vi "CLPT_Piezo_Solver.vi"() -> ()   [LabVIEW 2012]
uses:
  LEM_Params.ctl
panel:
  out "Displacement Ratio":dbl
  in  "Stop Button":bool
  in  "Constants.P":dbl=-500.0
  in  "Constants.Vac":dbl=-10.0
  out "LEM Parameters":T1
  out "error out":errorcluster
  out "XY Graph":cluster{"Radius":dbl[], "W(r)":dbl[]}(graph)
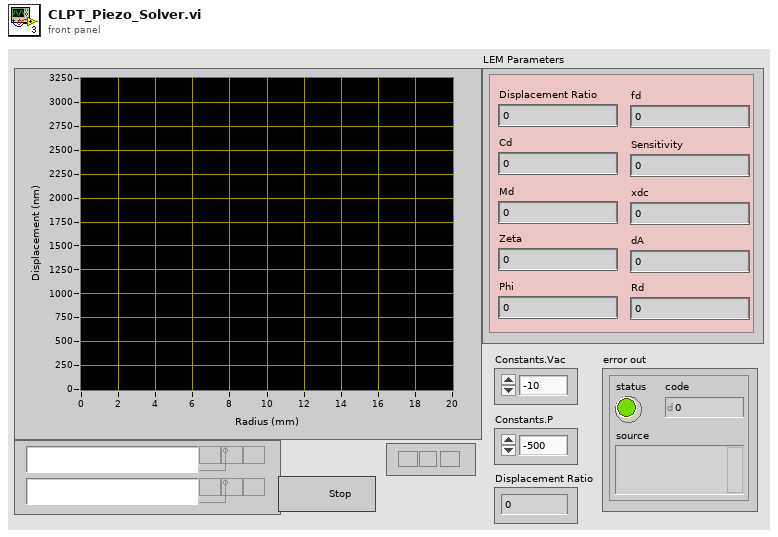
[diagram p1: front panel]
types:
  T1 = typedef "LEM_Params.ctl" = cluster{"Displacement Ratio":dbl, "Cd":dbl, "Md":dbl, "xdc":dbl, "fd":dbl, "Sensitivity":dbl, "dA":dbl, "Rd":dbl, "Zeta":dbl, "Phi":dbl}
  T2 = typedef "Model Data.ctl" = cluster{"Disc Properties":cluster{"Type":T3, "Disc Model":T4}, "Constants":cluster{"Radius":dbl[], "U(r)":dbl[], "W(r)":dbl[], "Vac":dbl, "P":dbl, "RiRo":dbl, "Area Density (r)":dbl[], "Ro":dbl, "Ri":dbl, "Z":dbl[], "Nr":dbl, "Mr":dbl, "c":dbl[], "AoC":dbl, "BoC":dbl, "AiC":dbl, "BiC":dbl, "f1":dbl, "f2":dbl}, "LEM Parameters":T1, "Layer Properties":T5[], "Matricies":T6}
  T3 = typedef "PZT type.ctl" = enum16{"Bimorph", "Unimorph"}
  T4 = typedef "Piezo_Discs.ctl" = enum16{"FTBD-21T-4.0A1", "PZT-5A (Gallas 1)", "PZT-5A (Gallas 2)", "AB4113B", "Create new disc...", "Load disc from file..."}
  T5 = typedef "Layer Properties.ctl" = cluster{"E":dbl, "R":dbl, "rho":dbl, "rhoA":dbl, "v":dbl, "A":dbl, "t":dbl, "d31":dbl, "size":enum16{"Outer", "Inner"}}
  T6 = typedef "Matricies.ctl" = cluster{"Aint":dbl[][], "Bint":dbl[][], "Dint":dbl[][], "Aout":dbl[][], "Bout":dbl[][], "Dout":dbl[][], "b":dbl[], "K":dbl[][]}
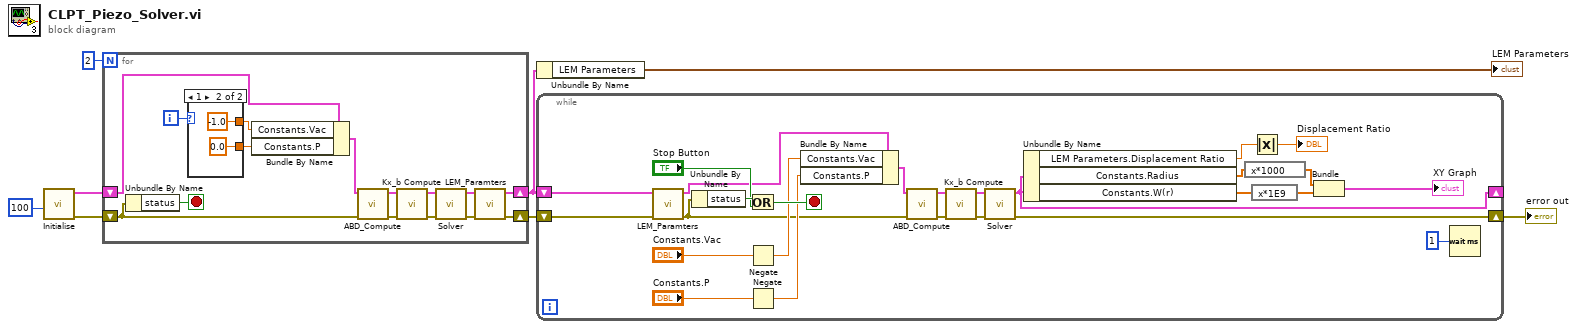
[diagram p0: block diagram]
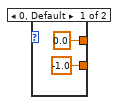
[diagram p2: hidden frame]
diagram:
  n1 = call "Initialise.vi"("Radial Points"=100) -> ("error out"=w5:errorcluster, "Model Data"=w7:T2)  [unwired: 9 in]
  n2 = for {
    N: 2 -> [_]
    shift-right: [w10] -> w2
    shift-left: w7 -> [w23]
    shift-right: [w15] -> w3
    shift-left: w5 -> [w9]
    i -> [w14]
    stop <- w11 stop-if-true
    n3 = Unbundle By Name(w9) -> ("status"=w11:bool)
    n4 = case shown="1" w14 {
      tunnel: [0.0 -1.0] -> w13
      tunnel: [-1.0 0.0] -> w12
      frame 0, Default {
      }
      frame 1 {
      }
    }
    n5 = Bundle By Name(cluster=w23, "Constants.Vac"=w13, "Constants.P"=w12) -> (w22:T2)
    n6 = call "ABD_Compute.vi"("error in"=w9, "Model Data"=w22) -> ("error out"=w21:errorcluster, "Model Data out"=w20:T2)  [unwired: 8 in]
    n7 = call "Kx_b Compute.vi"("error in"=w21, "Model Data"=w20) -> ("error out"=w19:errorcluster, "Model Data out"=w18:T2)  [unwired: 8 in]
    n8 = call "Solver.vi"("error in"=w19, "Model Data"=w18) -> ("error out"=w16:errorcluster, "Model Data out"=w17:T2)  [unwired: 8 in]
    n9 = call "LEM_Paramters.vi"("error in"=w16, "Model Data"=w17) -> ("error out"=w15:errorcluster, "Model Data Out"=w10:T2)  [unwired: 8 in]
  }
  n10 = Unbundle By Name(w2) -> ("LEM Parameters"=→"LEM Parameters":T1)
  n11 = while {
    shift-right: [w36] -> w4
    shift-left: w3 -> [w33]
    shift-right: [w43] -> _
    shift-left: w2 -> [w31]
    stop <- w39 stop-if-true
    n12 = call "LEM_Paramters.vi"("error in"=w33, "Model Data"=w31) -> ("error out"=w32:errorcluster, "Model Data Out"=w30:T2)  [unwired: 8 in]
    n13 = Unbundle By Name(w32) -> ("status"=w41:bool)
    n14 = Or(x=w41, y="Stop Button") -> (x .or. y?=w39:bool)
    n15 = Negate(x="Constants.Vac") -> (-x=w37:dbl)
    n16 = Negate(x="Constants.P") -> (-x=w38:dbl)
    n17 = Bundle By Name(cluster=w30, "Constants.Vac"=w37, "Constants.P"=w38) -> (w49:T2)
    n18 = call "ABD_Compute.vi"("error in"=w32, "Model Data"=w49) -> ("error out"=w50:errorcluster, "Model Data out"=w51:T2)  [unwired: 8 in]
    n19 = call "Kx_b Compute.vi"("error in"=w50, "Model Data"=w51) -> ("error out"=w52:errorcluster, "Model Data out"=w53:T2)  [unwired: 8 in]
    n20 = call "Solver.vi"("error in"=w52, "Model Data"=w53) -> ("error out"=w36:errorcluster, "Model Data out"=w43:T2)  [unwired: 8 in]
    n21 = Unbundle By Name(w43) -> ("LEM Parameters.Displacement Ratio"=w29:dbl, "Constants.Radius"=w46:dbl[], "Constants.W(r)"=w45:dbl[])
    n22 = expression code="x*1000"(w46) -> (w48:dbl[])
    n23 = Absolute Value(x=w29) -> (abs(x)=→"Displacement Ratio":dbl)
    n24 = expression code="x*1E9"(w45) -> (w47:dbl[])
    n25 = Bundle("Radius"=w48, "W(r)"=w47) -> (→"XY Graph":cluster{"Radius":dbl[], "W(r)":dbl[]})  [unwired: 1 in]
    n26 = Wait (ms)(milliseconds to wait=u32 1) -> ()  [unwired: 1 out]
  }
  "error out" <- w4
